vi "Chronos GUI Get Plots and Axes.vi"(8 "error in (no error)":errorcluster, 10 "Ch Data":T3[](array[typedef]), 11 "Select Ch":string[](array[string])) -> (0 "error out":errorcluster, 3 "Plot Map":T1)   [LabVIEW 2021]
uses:
  Viewer/cluster CC Channel from TDMS.ctl
  Chronos cluster Map Limit Plots.ctl
  typedefs/Chronos cluster Plot Data and Limits.ctl
panel:
  out "Plot Names":string[](array[string])
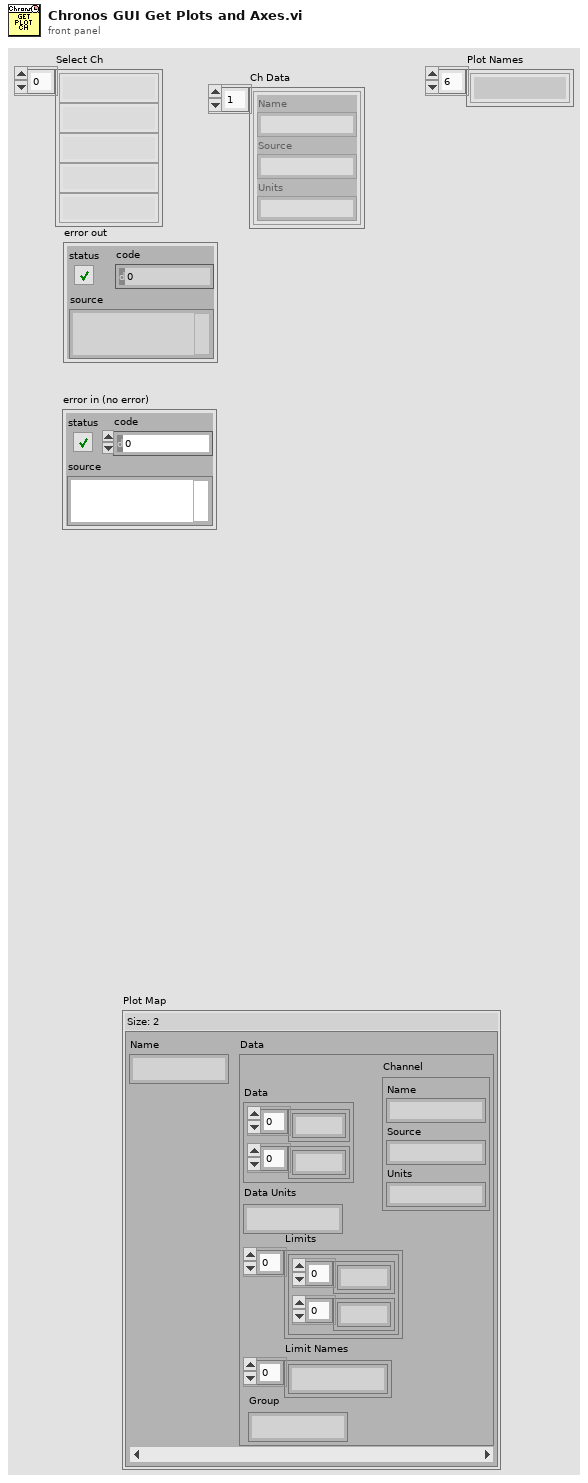
[diagram p1: front panel]
types:
  T1 = typedef "Chronos cluster Map Limit Plots.ctl" = map{string, T2}
  T2 = typedef "Chronos cluster Plot Data and Limits.ctl" = cluster{"Data":cluster{dbl[], dbl[]}, "Data Units":string, "Limits":cluster{dbl[], dbl[]}[], "Limit Names":string[], "Channel":T3, "Group":string}
  T3 = typedef "cluster CC Channel from TDMS.ctl" = cluster{"Name":string, "Source":string, "Units":string}
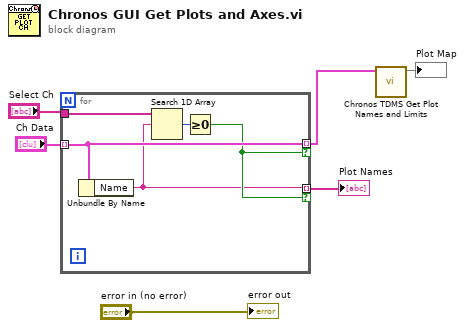
[diagram p0: block diagram]
diagram:
  n1 = for {
    tunnel: "Select Ch" -> [w11]
    tunnel: "Ch Data" -> [w9] mode=indexing
    tunnel: [w9] -> w2 mode=indexing if=w8
    tunnel: [w7] -> w4 mode=indexing if=w8
    n2 = Unbundle By Name(w9) -> ("Name"=w7:string)
    n3 = Search 1D Array(1D array=w11, element=w7) -> (index of element=w10:i32)  [unwired: 1 in]
    n4 = Greater Or Equal To 0?(x=w10) -> (x >= 0?=w8:bool)
  }
  "Plot Names" <- w4
  n5 = call "Chronos TDMS Get Plot Names and Limits.vi"("Ch Data"=w2) -> ("Limit Plot Map"=→"Plot Map":T1)  [unwired: 9 in, 1 out]
  "error out" <- "error in (no error)"
